vi "SubTestEConv.vi"() -> ()   [LabVIEW 2019]
panel:
  out "lambda m":dbl format="%#_6p"
  out "delta bd m":dbl format="%#_6p"
  out "Conv/BEnergy (eV)":dbl caption="Energy :" format="%#_6p"
  out "Conv/BTime (s)":dbl caption="Time :" format="%#_6p"
  out "Conv/BFreq (Hz)":dbl caption="Frequency :" format="%#_6p"
  out "Conv/BWavelength (nm)":dbl caption="Wavelength :" format="%#_6p"
  in  "Conv/DBunit Loc In":u16(ring) items=["eV", "m"]
  in  "Conv/Bandwidth In Loc":dbl format="%#_6p"
  in  "Conv/Bandwidth unit In":u16(ring) items=["eV", "m", "s", "Hz"]
  in  "Conv/Bandwidth In":dbl format="%#_6p"
  # "BD"
  # "@"
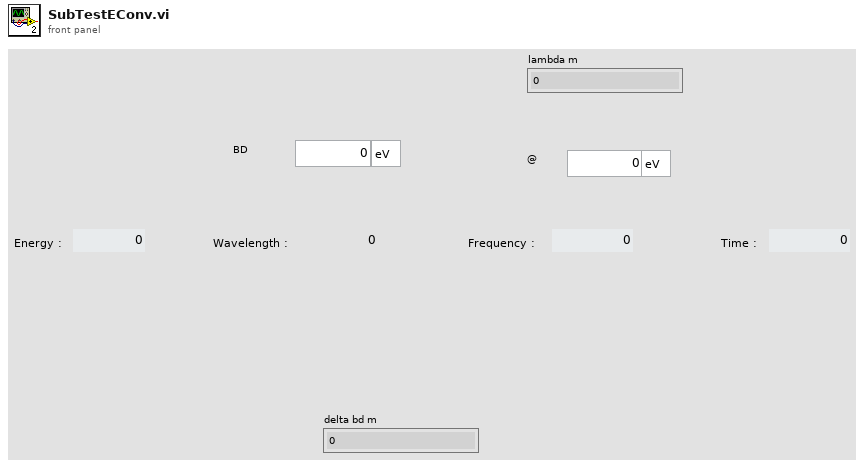
[diagram p1: front panel]
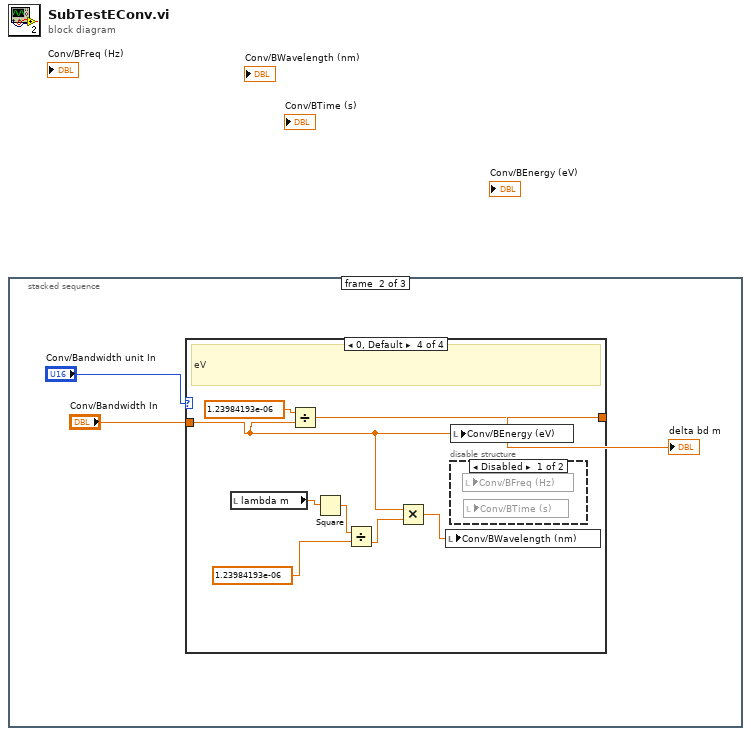
[diagram p0: block diagram]
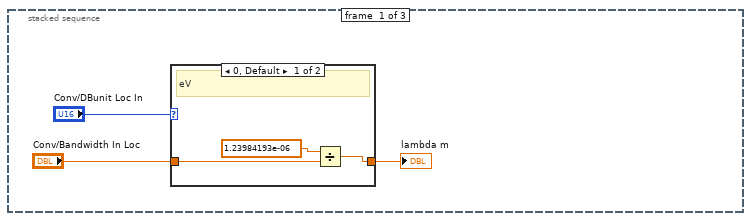
[diagram p2: hidden frame]
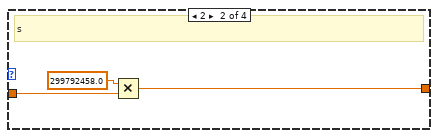
[diagram p5: hidden frame]
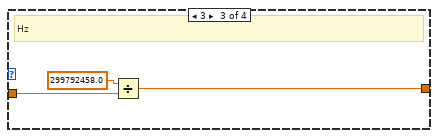
[diagram p6: hidden frame]
diagram:
  n1 = stacked-sequence {
    frame #0 {
      n2 = case shown="0, Default" "Conv/DBunit Loc In" {
        tunnel: "Conv/Bandwidth In Loc" -> [w5 w7]
        tunnel: [w4 w7] -> w1
        frame 0, Default {
          # "eV"
          n3 = Divide(x=1.23984193e-06, y=w5) -> (x/y=w4:dbl)
        }
        frame 1 {
          # "m"
        }
      }
      "lambda m" <- w1
    }
    frame #1 {
      n4 = case shown="0, Default" "Conv/Bandwidth unit In" {
        tunnel: "Conv/Bandwidth In" -> [w11 w13 w16 w18]
        tunnel: [w11 w12 w15 w24] -> w10
        frame 1 {
          # "m"
        }
        frame 2 {
          # "s"
          n5 = Multiply(x=299792458.0, y=w13) -> (x*y=w12:dbl)
        }
        frame 3 {
          # "Hz"
          n6 = Divide(x=299792458.0, y=w16) -> (x/y=w15:dbl)
        }
        frame 0, Default {
          # "eV"
          n7 = local read "lambda m"() -> (w23:dbl)
          n8 = Divide(x=1.23984193e-06, y=w18) -> (x/y=w24:dbl)
          n9 = Square(x=w23) -> (x^2=w22:dbl)
          n10 = Divide(x=w22, y=1.23984193e-06) -> (x/y=w20:dbl)
          n11 = Multiply(x=w18, y=w20) -> (x*y=w19:dbl)
          n12 = local write "Conv/BWavelength (nm)"(w19) -> ()
          n13 = local write "Conv/BEnergy (eV)"(w18) -> ()
          n14 = disable-structure shown="Disabled" {
            frame Disabled {
              n15 = local read "Conv/BFreq (Hz)"() -> ()  [unwired: 1 in]
              n16 = local read "Conv/BTime (s)"() -> ()  [unwired: 1 in]
            }
            frame Enabled {
            }
          }
        }
      }
      "delta bd m" <- w10
    }
    frame #2 {
      # "Convert from wavelength at wavelength to all"
    }
  }
